vi "Marker Search.vi"(5 "Marker (1)":i32=1, 7 "Channel (1)":i32=1, 8 "error in (no error)":errorcluster, 10 "Function (0: Maximum)":u16(ring) items=["Maximum", "Minimum", "Peak", "Left Peak", "Right Peak", "Target", "Left Target", "Right Target"], 11 "VISA resource name":refnum<visa-resource-name>) -> (0 "error out":errorcluster, 1 "Y Primary Value":dbl format="%^.2e", 2 "X Value":dbl format="%^.2e", 3 "VISA resource name out":refnum<visa-resource-name>, 4 "Y Secondary Value":dbl format="%^.2e")   [LabVIEW 2011, in "Agilent ENA Series.lvlib"]
doc: "This VI searches marker and returns position and value of founded marker."
uses:
  Agilent ENA Series.lvlib
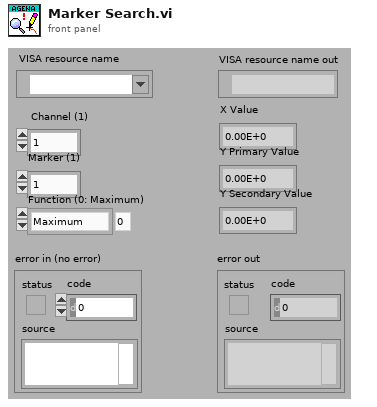
[diagram p1: front panel]
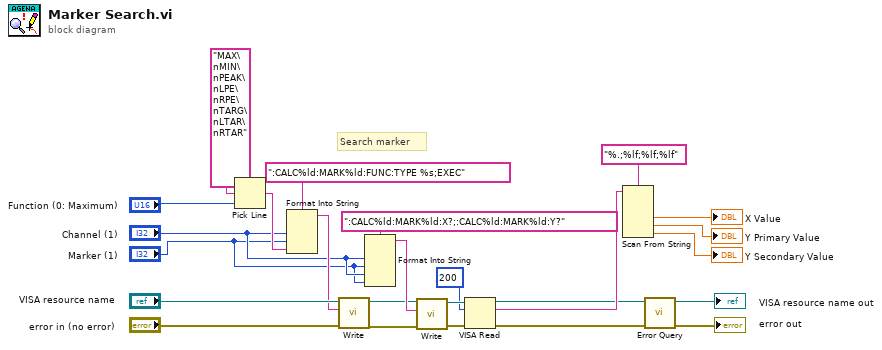
[diagram p0: block diagram]
diagram:
  # "Search marker"
  n1 = Pick Line(multi-line string="MAX\nMIN\nPEAK\nLPE\nRPE\nTARG\nLTAR\nRTAR", line index="Function (0: Maximum)") -> (output string=w19:string)  [unwired: 1 in]
  n2 = Format Into String(format string=":CALC%ld:MARK%ld:FUNC:TYPE %s;EXEC", "Channel (1)", "Marker (1)", w19) -> (resulting string=w22:string)  [unwired: 2 in, 1 out]
  n3 = call "Write.vi"("error in (no error)"="error in (no error)", "String ()"=w22, "VISA resource name"="VISA resource name") -> ("error out"=w13:errorcluster, "VISA resource name out"=w14:refnum<visa-resource-name>)  [unwired: 6 in, 1 out]
  n4 = Format Into String(format string=":CALC%ld:MARK%ld:X?;:CALC%ld:MARK%ld:Y?", "Channel (1)", "Marker (1)", "Channel (1)", "Marker (1)") -> (resulting string=w18:string)  [unwired: 2 in, 1 out]
  n5 = call "Write.vi"("error in (no error)"=w13, "String ()"=w18, "VISA resource name"=w14) -> ("error out"=w11:errorcluster, "VISA resource name out"=w12:refnum<visa-resource-name>)  [unwired: 6 in, 1 out]
  n6 = VISA Read(VISA resource name=w12, byte count=u32 200, error in (no error)=w11) -> (VISA resource name out=w4:refnum<visa-resource-name>, read buffer=w6:string, error out=w3:errorcluster)  [unwired: 1 out]
  n7 = Scan From String(format string="%.;%lf;%lf;%lf", input string=w6) -> (output 1=→"X Value":dbl, output 2=→"Y Primary Value":dbl, output 3=→"Y Secondary Value":dbl)  [unwired: 5 in, 3 out]
  n8 = call "Error Query.vi"("error in (no error)"=w3, "VISA resource name"=w4) -> ("error out"=→"error out":errorcluster, "VISA resource name out"=→"VISA resource name out":refnum<visa-resource-name>)  [unwired: 6 in, 2 out]
